vi "VariantAttributeReadExample.vi"() -> ()   [LabVIEW 2014, in "examples.lvlib"]
uses:
  vis/tango_vi.llb/_TangoState_t.ctl
  vis/tango_vi.llb/_TangoReadAttributeVariant.vi
  examples.lvlib
  vis/tango_vi.llb/tango.lvlib
panel:
  out "sys/database/2:State":T1
  out "sys/database/2:Status":string
  out "sys/database/2:Timing_info":string[](array[string])
  out "sys/database/2:Timing_index":string[](array[string])
  out "sys/database/2:Timing_calls":dbl[](array[numeric])
  out "sys/database/2:Timing_maximum":dbl[](array[numeric])
  out "sys/database/2:Timing_minimum":dbl[](array[numeric])
  out "sys/database/2:Timing_average":dbl[](array[numeric])
  out "sys/database/2:StoredProcedureRelease":string
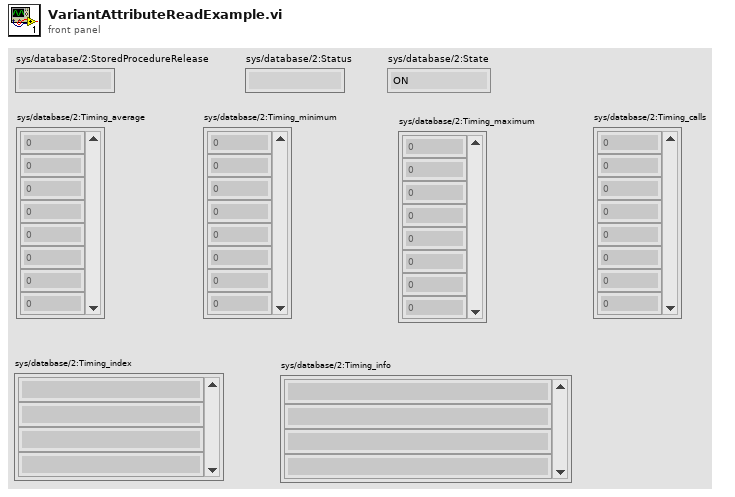
[diagram p1: front panel]
types:
  T1 = typedef "tango.lvlib/_TangoState_t.ctl" = enum32{"ON", "OFF", "CLOSE", "OPEN", "INSERT", "EXTRACT", "MOVING", "STANDBY", "FAULT", "INIT", "RUNNING", "ALARM", "DISABLE", "UNKNOWN"}
  T2 = enum8{"Enabled", "Disabled", "Disabled and Grayed Out"}
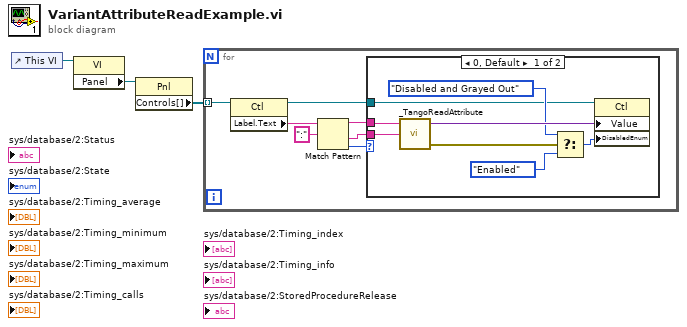
[diagram p0: block diagram]
diagram:
  n1 = control-ref of="This VI"() -> (w3:refnum<vi>)
  n2 = property class="VI"(reference=w3) -> ("Panel"=w2:refnum<vi>)  [unwired: 1 in, 2 out]
  n3 = property class="Pnl"(reference=w2) -> ("Controls[]"=w1:refnum<vi>[])  [unwired: 1 in, 2 out]
  n4 = for {
    tunnel: w1 -> [w10] mode=indexing
    n5 = property class="Ctl"(reference=w10) -> (reference out=w6:refnum<vi>, "Label.Text"=w7:string)  [unwired: 1 in, 1 out]
    n6 = Match Pattern(string=w7, regular expression=":") -> (before substring=w5:string, after substring=w4:string, offset past match=w8:i32)  [unwired: 1 in, 1 out]
    n7 = case shown="0, Default" w8 {
      tunnel: w6 -> [w11 _]
      tunnel: w5 -> [w13 _]
      tunnel: w4 -> [w12 _]
      frame 0, Default {
        n8 = call-poly "_TangoReadAttribute.vi"("attribute name"=w12, "device name"=w13) -> ("error out"=w17:errorcluster, "value"=w18:variant)  [unwired: 1 in, 1 out]
        n9 = Select(t=T2."Disabled and Grayed Out", s=w17, f=T2."Enabled" ("Disabled")) -> (s? t:f=w16:T2)
        n10 = property class="Ctl"(reference=w11, "Value"=w18, "DisabledEnum"=w16) -> ()  [unwired: 1 in, 2 out]
      }
      frame -1 {
      }
    }
  }
